vi "468_lab8_noise_sim.vi"(4 "duration":dbl=1.0, 5 "fs":dbl=360.0, 6 "noise amp":dbl=0.2 step=0.1, 7 "noise type":T1(ring)) -> (3 "noise":dbl[](graph))   [LabVIEW 2025]
uses:
  <vilib>/Analysis/4window.llb/Flat Top Window (DBL).vi
  <vilib>/Analysis/4window.llb/AllCosWindow (DBL).vi
  <vilib>/Analysis/NI_AALBase.lvlib
  <vilib>/Analysis/NI_AALPro.lvlib
panel:
  out "length":i32
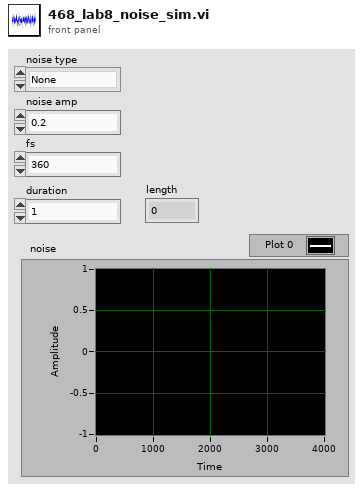
[diagram p1: front panel]
types:
  T1 = enum16{"None", "Slow Drift", "White noise", "Muscle artifact", "Motion artifact", "60 Hz"}
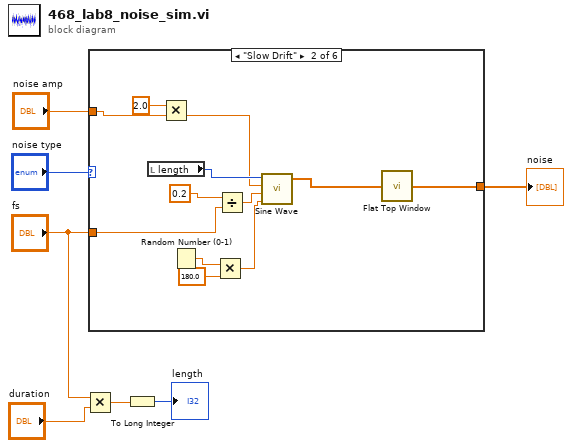
[diagram p0: block diagram]
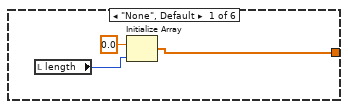
[diagram p2: hidden frame]
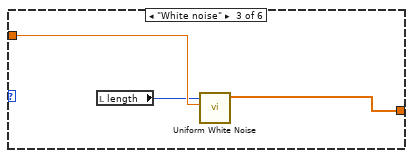
[diagram p3: hidden frame]
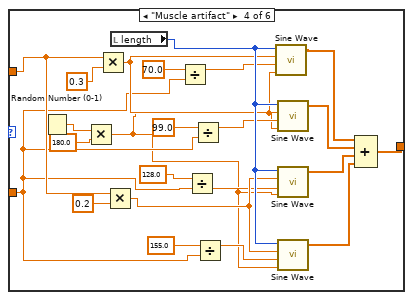
[diagram p4: hidden frame]
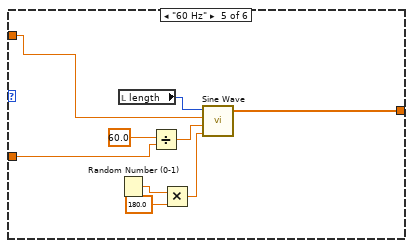
[diagram p5: hidden frame]
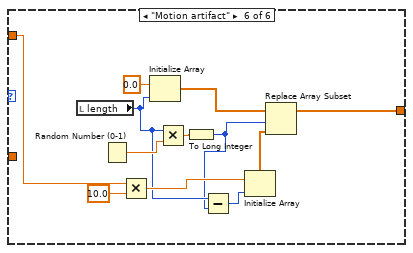
[diagram p6: hidden frame]
diagram:
  n1 = Multiply(x="fs", y="duration") -> (x*y=w2:dbl)
  n2 = case shown="\"Slow Drift\"" "noise type" {
    tunnel: "noise amp" -> [_ w22 w25 w47 w57 w66]
    tunnel: "fs" -> [_ w18 _ w29 w53 _]
    tunnel: [w8 w16 w23 w35 w55 w63] -> w5
    frame "None", Default {
      n3 = local read "length"() -> (w9:i32)
      n4 = Initialize Array(0.0 ("element"), w9) -> (w8:dbl[])
    }
    frame "Slow Drift" {
      n5 = local read "length"() -> (w21:i32)
      n6 = Multiply(x=2.0, y=w22) -> (x*y=w12:dbl)
      n7 = Random Number (0-1)() -> (number: 0 to 1=w15:dbl)
      n8 = Multiply(x=w15, y=180.0) -> (x*y=w13:dbl)
      n9 = Divide(x=0.2 ("frequency"), y=w18) -> (x/y=w17:dbl)
      n10 = call <vilib>:"Sine Wave.vi"("samples"=w21, "amplitude"=w12, "frequency"=w17, "phase in"=w13) -> ("sine wave"=w20:dbl[])  [unwired: 1 in, 2 out]
      n11 = call-poly <vilib>:"Flat Top Window.vi"("X"=w20) -> ("Windowed X"=w16:dbl[])  [unwired: 1 out]
    }
    frame "White noise" {
      n12 = local read "length"() -> (w24:i32)
      n13 = call <vilib>:"Uniform White Noise.vi"("amplitude"=w25, "samples"=w24) -> ("uniform white noise"=w23:dbl[])  [unwired: 8 in, 1 out]
    }
    frame "Muscle artifact" {
      n14 = Random Number (0-1)() -> (number: 0 to 1=w28:dbl)
      n15 = Multiply(x=w28, y=180.0) -> (x*y=w26:dbl)
      n16 = Multiply(x=w47, y=0.3) -> (x*y=w40:dbl)
      n17 = Multiply(x=w47, y=0.2) -> (x*y=w43:dbl)
      n18 = local read "length"() -> (w45:i32)
      n19 = Divide(x=70.0 ("frequency"), y=w29) -> (x/y=w34:dbl)
      n20 = Divide(x=128.0 ("frequency"), y=w29) -> (x/y=w32:dbl)
      n21 = Divide(x=99.0 ("frequency"), y=w29) -> (x/y=w33:dbl)
      n22 = Divide(x=155.0 ("frequency"), y=w29) -> (x/y=w30:dbl)
      n23 = call <vilib>:"Sine Wave.vi"("samples"=w45, "amplitude"=w40, "frequency"=w34, "phase in"=w26) -> ("sine wave"=w39:dbl[])  [unwired: 1 in, 2 out]
      n24 = call <vilib>:"Sine Wave.vi"("samples"=w45, "amplitude"=w40, "frequency"=w33, "phase in"=w26) -> ("sine wave"=w38:dbl[])  [unwired: 1 in, 2 out]
      n25 = call <vilib>:"Sine Wave.vi"("samples"=w45, "amplitude"=w43, "frequency"=w32, "phase in"=w26) -> ("sine wave"=w37:dbl[])  [unwired: 1 in, 2 out]
      n26 = call <vilib>:"Sine Wave.vi"("samples"=w45, "amplitude"=w43, "frequency"=w30, "phase in"=w26) -> ("sine wave"=w36:dbl[])  [unwired: 1 in, 2 out]
      n27 = Compound Arithmetic op=ADD(w39, w38, w37, w36) -> (w35:dbl[])
    }
    frame "60 Hz" {
      n28 = Random Number (0-1)() -> (number: 0 to 1=w51:dbl)
      n29 = local read "length"() -> (w56:i32)
      n30 = Divide(x=60.0 ("frequency"), y=w53) -> (x/y=w52:dbl)
      n31 = Multiply(x=w51, y=180.0) -> (x*y=w49:dbl)
      n32 = call <vilib>:"Sine Wave.vi"("samples"=w56, "amplitude"=w57, "frequency"=w52, "phase in"=w49) -> ("sine wave"=w55:dbl[])  [unwired: 1 in, 2 out]
    }
    frame "Motion artifact" {
      n33 = local read "length"() -> (w59:i32)
      n34 = Random Number (0-1)() -> (number: 0 to 1=w67:dbl)
      n35 = Multiply(x=w66, y=10.0) -> (x*y=w62:dbl)
      n36 = Initialize Array(0.0 ("element"), w59) -> (w68:dbl[])
      n37 = Multiply(x=w59, y=w67) -> (x*y=w64:dbl)
      n38 = To Long Integer(number=w64) -> (32bit integer=w58:i32)
      n39 = Subtract(x=w59, y=w58) -> (x-y=w60:i32)
      n40 = Initialize Array(w62, w60) -> (w61:dbl[])
      n41 = Replace Array Subset(array=w68, new element=w61, index=w58) -> (w63:dbl[])
    }
  }
  "noise" <- w5
  n42 = To Long Integer(number=w2) -> (32bit integer=→"length":i32)
